vi "Read Discrete Inputs.vi"(7 "unit ID":u8, 8 "error in":errorcluster, 9 "number of inputs":u16, 10 "starting address":u16, 11 "Modbus master in":refnum<class "Modbus Master.lvclass">) -> (0 "error out":errorcluster, 2 "discrete inputs":bool[](array[boolean]), 3 "Modbus master out":refnum<class "Modbus Master.lvclass">)   [LabVIEW 2013, in "Modbus Library - Advance.lvlib" / "Modbus Master.lvclass"]
doc: "Reads <B>number of inputs</B> discrete inputs starting at <B>starting address</B> from the device."
uses:
  Modbus Master.lvclass
  Modbus Master.lvclass/Modbus Master.ctl
  Modbus API.lvclass/Modbus API.ctl
  Transmission Data Unit/Transmission Data Unit.lvclass/Transmission Data Unit.ctl
  Transmission Data Unit/Transmission Data Unit.lvclass
  Modbus API.lvclass
  Master Function Definition/Master Function Definition.lvclass
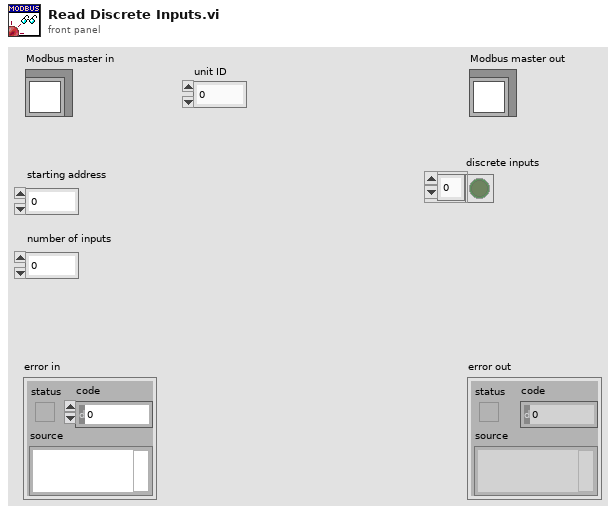
[diagram p1: front panel]
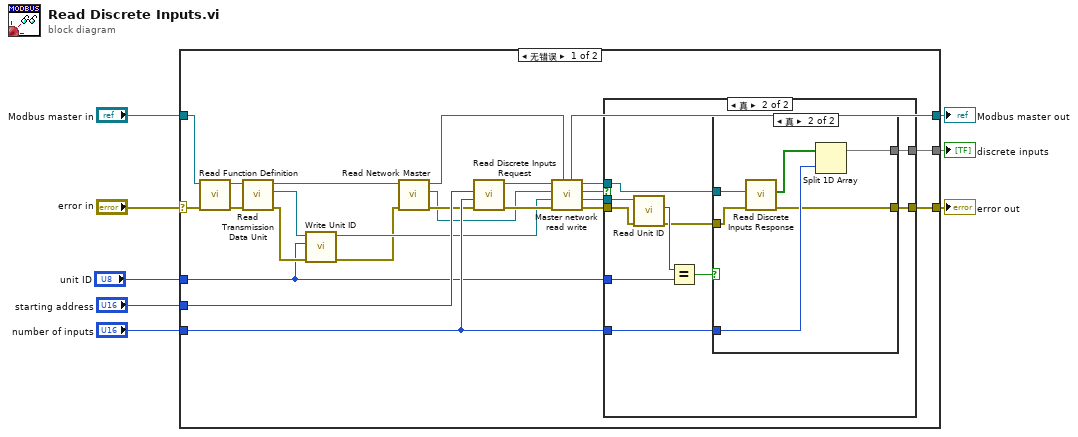
[diagram p0: block diagram]
diagram:
  n1 = case shown="无错误" "error in" {
    selector: "error in" -> [w20 w51]
    tunnel: "Modbus master in" -> [w17 w52]
    tunnel: [w24 w52] -> w7
    tunnel: [w25 w51] -> w6
    tunnel: [w30 _] -> w4
    tunnel: "number of inputs" -> [w29 _]
    tunnel: "starting address" -> [w31 _]
    tunnel: "unit ID" -> [w9 _]
    frame No Error {
      n2 = call "Read Function Definition.vi"("error in"=w20, "Modbus master in"=w17) -> ("error out"=w22:errorcluster, "Modbus master out"=w21:refnum<class "Modbus Master.lvclass">)  [unwired: 7 in, 1 out]
      n3 = call "Read Transmission Data Unit.vi"("error in"=w22, "Modbus instance in"=w21) -> ("error out"=w13:errorcluster, "transmission data unit"=w14:refnum<class "Transmission Data Unit.lvclass">, "Modbus instance out"=w23:refnum<class "Modbus Master.lvclass">)  [unwired: 7 in]
      n4 = call "Write Unit ID.vi"("error in"=w13, "unit ID"=w9, "transmission data unit in"=w14) -> ("error out"=w11:errorcluster, "transmission data unit out"=w12:refnum<class "Transmission Data Unit.lvclass">)  [unwired: 7 in]
      n5 = call "Read Network Master.vi"("error in"=w11, "Modbus master in"=w23) -> ("error out"=w19:errorcluster, "network master"=w16:refnum<class "Network Master.lvclass">, "Modbus master out"=w18:refnum<class "Modbus Master.lvclass">)  [unwired: 7 in]
      n6 = call "Read Discrete Inputs Request.vi"("error in"=w19, "Number of inputs"=w29, "starting address"=w31) -> ("error out"=w32:errorcluster, "modbus data unit out"=w27:refnum<class "Modbus Data Unit.lvclass">)  [unwired: 7 in]
      n7 = call "Master network read write.vi"("Modbus master in"=w18, "error in"=w32, "transmission data unit in"=w12, "network master in"=w16, "Modbus data unit in"=w27) -> ("error out"=w28:errorcluster, "transmission data unit out"=w10:refnum<class "Transmission Data Unit.lvclass">, "PDU Valid?"=w15:bool, "Modbus data unit out"=w26:refnum<class "Modbus Data Unit.lvclass">, "Modbus master out"=w24:refnum<class "Modbus Master.lvclass">)  [unwired: 2 in]
      n8 = case shown="真" w15 {
        tunnel: [_ w43] -> w30
        tunnel: w29 -> [_ w42]
        tunnel: w28 -> [w33 w38]
        tunnel: w26 -> [_ w41]
        tunnel: [w33 w40] -> w25
        tunnel: w10 -> [_ w39]
        tunnel: w9 -> [_ w36]
        frame False {
        }
        frame True {
          n9 = call "Read Unit ID.vi"("error in"=w38, "transmission data unit in"=w39) -> ("error out"=w35:errorcluster, "unit ID"=w37:u8)  [unwired: 7 in, 1 out]
          n10 = Equal?(x=w37, y=w36) -> (x = y?=w34:bool)
          n11 = case shown="真" w34 {
            tunnel: [_ w49] -> w43
            tunnel: w42 -> [_ w48]
            tunnel: w41 -> [_ w47]
            tunnel: [w44 w46] -> w40
            tunnel: w35 -> [w44 w45]
            frame False {
            }
            frame True {
              n12 = call "Read Discrete Inputs Response.vi"("error in"=w45, "modbus data unit in"=w47) -> ("error out"=w46:errorcluster, "Data"=w50:bool[])  [unwired: 8 in]
              n13 = Split 1D Array(array=w50, index=w48) -> (first subarray=w49:bool[])  [unwired: 1 out]
            }
          }
        }
      }
    }
    frame Error {
    }
  }
  "error out" <- w6
  "Modbus master out" <- w7
  "discrete inputs" <- w4
